vi "PathSettings.vi"(11 "notifier":refnum<notifier>) -> ()   [LabVIEW 2013, in "main.lvlib"]
uses:
  main.lvlib
  Controls/Enum User Events.ctl
  Controls/Enum Save Action Events.ctl
  Globals/DataPathGlobalVariable.vi
panel:
  in  "Journal Template":path caption="Graf destination"
  in  "Graf destination":path
  in  "ReportFolder":path caption="Journal destination"
  in  "FolderPath":path caption="Data destination"
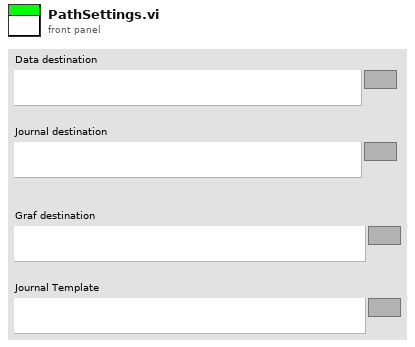
[diagram p1: front panel]
types:
  T1 = typedef "main.lvlib/Enum Save Action Events.ctl" = enum16{"LoadReportPath", "SaveReportPath", "Load Graph Path", "Save Graph Path", "LoadDataPath", "SaveDataPath", "Load Template Path", "Save Template Path", "Load PressureFactor", "Save PressureFactor", "Init", "Load Listbox", "Save Listbox", "LoadHospInfo", "SaveHospInfo", "Load DICOM Activation", "Save DICOM Activation", "LoadDICOMInfoWL", "SaveDICOMInfoWL", "LoadDICOMInfoPACS", "SaveDICOMInfoPACS", "Load ArmCalcMethod", "Save ArmCalcMethod", "LoadItemTags", "SaveItemTags", "LoadDICOMEncoding", "SaveDICOMEncoding", "LoadJournalType", "SaveJournalType", "LoadAcqFilterType", "SaveAcqFilterType", "Load Sequence", "Save Sequence", "Load Acquisition Mode", "Save Acquisition Mode", "Load General Settings", "Save General Settings", "Load Language", "Save Language", "Load Dicom Tags", "Save Dicom Tags", "Load BT Serial", "Save BT Serial", "Load BT License", "Save BT License"}
  T2 = typedef "main.lvlib/Enum User Events.ctl" = enum16{"User Event", "Init"}
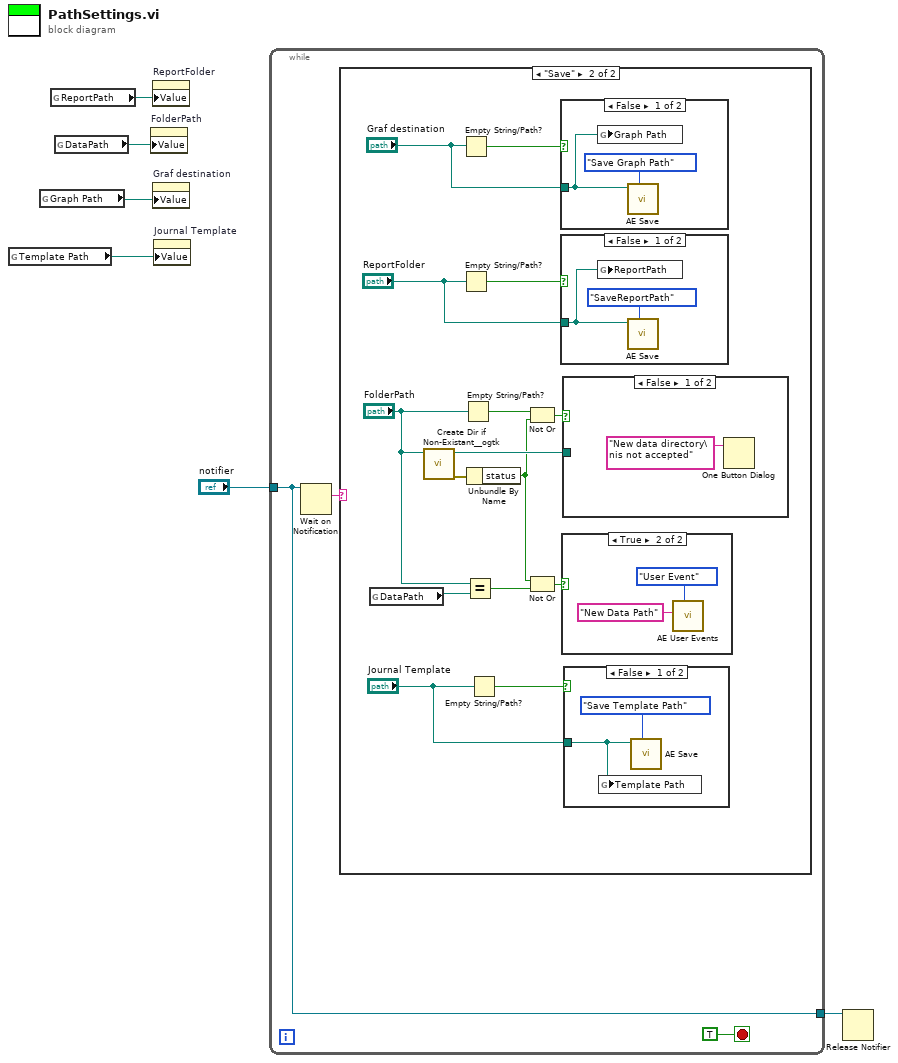
[diagram p0: block diagram]
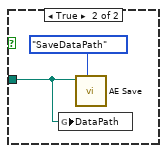
[diagram p7: hidden frame]
diagram:
  n1 = global read "DataPathGlobalVariable.vi" "Template Path"() -> (w1:path)
  n2 = global read "DataPathGlobalVariable.vi" "Graph Path"() -> (w2:path)
  n3 = global read "DataPathGlobalVariable.vi" "ReportPath"() -> (w4:path)
  n4 = global read "DataPathGlobalVariable.vi" "DataPath"() -> (w5:path)
  n5 = property on="FolderPath" class="Path"("Value"=w5) -> ()  [unwired: 2 in, 2 out]
  n6 = property on="ReportFolder" class="Path"("Value"=w4) -> ()  [unwired: 2 in, 2 out]
  n7 = property on="Graf destination" class="Path"("Value"=w2) -> ()  [unwired: 2 in, 2 out]
  n8 = property on="Journal Template" class="Path"("Value"=w1) -> ()  [unwired: 2 in, 2 out]
  n9 = while {
    tunnel: "notifier" -> [w7]
    tunnel: [w7] -> w3
    stop <- TRUE stop-if-true
    n10 = Wait on Notification(notifier=w7) -> (notification=w9:string)  [unwired: 3 in, 3 out]
    n11 = case shown="\"Save\"" w9 {
      frame "Cancel", Default {
      }
      frame "Save" {
        n12 = global read "DataPathGlobalVariable.vi" "DataPath"() -> (w20:path)
        n13 = call <userlib>:"Create Dir if Non-Existant__ogtk.vi"("Directory Path"="FolderPath") -> ("error out"=w15:errorcluster, "dup Directory Path"=w17:path)  [unwired: 8 in, 1 out]
        n14 = Empty String/Path?(string/path="Graf destination") -> (empty?=w23:bool)
        n15 = Empty String/Path?(string/path="ReportFolder") -> (empty?=w24:bool)
        n16 = Empty String/Path?(string/path="FolderPath") -> (empty?=w13:bool)
        n17 = Equal?(x="FolderPath", y=w20) -> (x = y?=w12:bool)
        n18 = Unbundle By Name(w15) -> ("status"=w11:bool)
        n19 = Empty String/Path?(string/path="Journal Template") -> (empty?=w19:bool)
        n20 = Not Or(1:w11, 2:w13) -> (0:w14:bool)
        n21 = Not Or(1:w12, 2:w11) -> (0:w10:bool)
        n22 = case shown="False" w23 {
          tunnel: "Graf destination" -> [w29 _]
          frame False {
            n23 = global write "DataPathGlobalVariable.vi" "Graph Path"(w29) -> ()
            n24 = call "AE Save.vi"("Variant In"=w29, "Action"=Enum_Save_Action_Events."Save Graph Path") -> ()  [unwired: 7 in, 2 out]
          }
          frame True {
          }
        }
        n25 = case shown="False" w24 {
          tunnel: "ReportFolder" -> [w31 _]
          frame False {
            n26 = global write "DataPathGlobalVariable.vi" "ReportPath"(w31) -> ()
            n27 = call "AE Save.vi"("Variant In"=w31, "Action"=Enum_Save_Action_Events."SaveReportPath") -> ()  [unwired: 7 in, 2 out]
          }
          frame True {
          }
        }
        n28 = case shown="True" w10 {
          frame False {
          }
          frame True {
            n29 = call "AE User Events.vi"("Action"=Enum_User_Events."User Event", "User Event"="New Data Path") -> ()  [unwired: 8 in, 2 out]
          }
        }
        n30 = case shown="False" w14 {
          tunnel: w17 -> [_ w34]
          frame False {
            n31 = One Button Dialog(message="New data directory\nis not accepted") -> ()  [unwired: 1 in, 1 out]
          }
          frame True {
            n32 = global write "DataPathGlobalVariable.vi" "DataPath"(w34) -> ()
            n33 = call "AE Save.vi"("Variant In"=w34, "Action"=Enum_Save_Action_Events."SaveDataPath") -> ()  [unwired: 7 in, 2 out]
          }
        }
        n34 = case shown="False" w19 {
          tunnel: "Journal Template" -> [w25 _]
          frame False {
            n35 = global write "DataPathGlobalVariable.vi" "Template Path"(w25) -> ()
            n36 = call "AE Save.vi"("Variant In"=w25, "Action"=Enum_Save_Action_Events."Save Template Path") -> ()  [unwired: 7 in, 2 out]
          }
          frame True {
          }
        }
      }
    }
  }
  n37 = Release Notifier(notifier=w3) -> ()  [unwired: 2 in, 3 out]
